vi "Param.vi"() -> ()   [LabVIEW 2015]
uses:
  Variable globale.vi
panel:
  in  "Decel":dbl
  in  "Accel":dbl
  in  "stop":bool
  in  "Ressolution Codeur":dbl
  in  "Diametre Galet Codeur":dbl
  in  "Diametre Plateau":dbl
  in  "Decel Max":dbl
  in  "Accel Max":dbl
  in  "Vitesse Max":dbl
  # "PARAMETRES UTILISATEUR"
  # "mm/s²"
  # "mm/s²"
  # "PARAMETRES SYSTEME"
  # "mm/s"
  # "mm"
  # "mm/s²"
  # "mm"
  # "mm/s²"
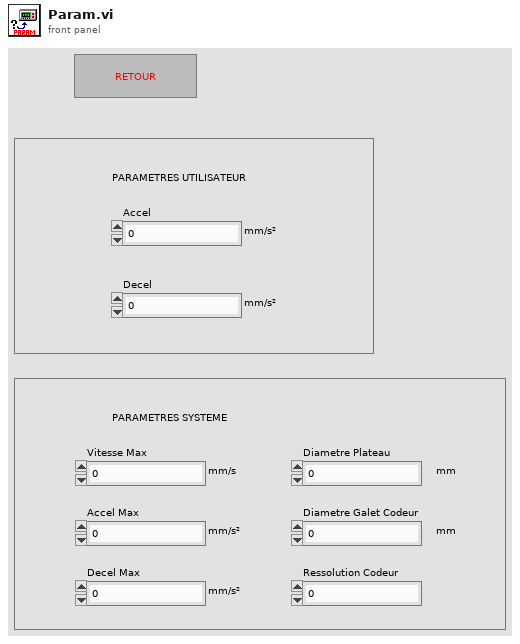
[diagram p1: front panel]
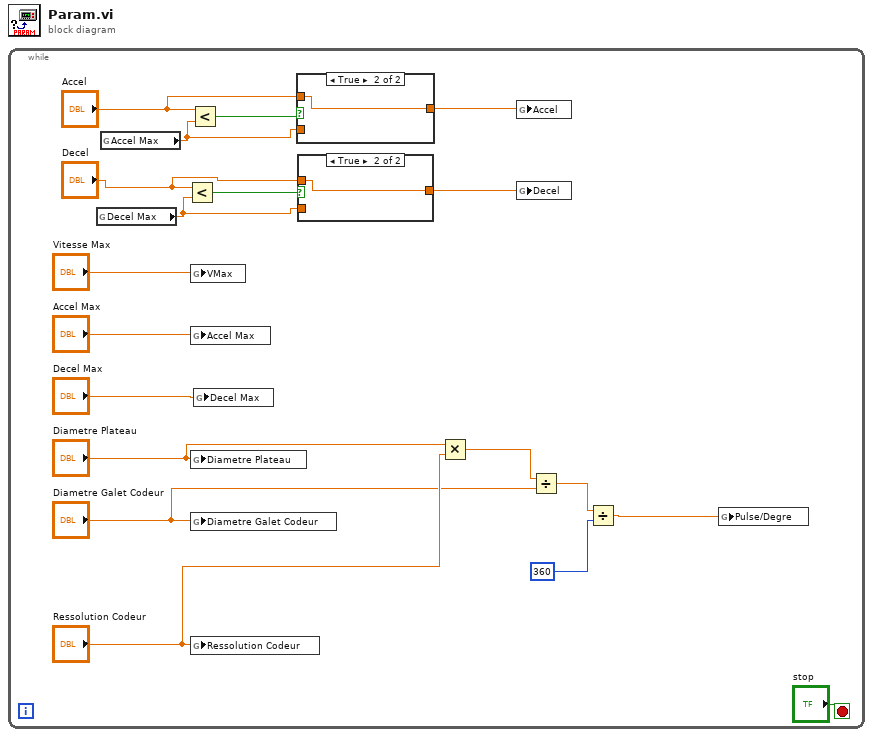
[diagram p0: block diagram]
diagram:
  n1 = while {
    stop <- "stop" stop-if-true
    n2 = global read "Variable globale.vi" "Decel Max"() -> (w2:dbl)
    n3 = global read "Variable globale.vi" "Accel Max"() -> (w6:dbl)
    n4 = Less?(x="Decel", y=w2) -> (x < y?=w4:bool)
    n5 = Less?(x="Accel", y=w6) -> (x < y?=w8:bool)
    n6 = global write "Variable globale.vi" "VMax"("Vitesse Max") -> ()
    n7 = global write "Variable globale.vi" "Accel Max"("Accel Max") -> ()
    n8 = global write "Variable globale.vi" "Diametre Plateau"("Diametre Plateau") -> ()
    n9 = global write "Variable globale.vi" "Diametre Galet Codeur"("Diametre Galet Codeur") -> ()
    n10 = global write "Variable globale.vi" "Ressolution Codeur"("Ressolution Codeur") -> ()
    n11 = global write "Variable globale.vi" "Decel Max"("Decel Max") -> ()
    n12 = case shown="True" w8 {
      tunnel: "Accel" -> [_ w23]
      tunnel: w6 -> [w22 _]
      tunnel: [w22 w23] -> w5
      frame False {
      }
      frame True {
      }
    }
    n13 = case shown="True" w4 {
      tunnel: "Decel" -> [_ w21]
      tunnel: w2 -> [w20 _]
      tunnel: [w20 w21] -> w1
      frame False {
      }
      frame True {
      }
    }
    n14 = Multiply(x="Diametre Plateau", y="Ressolution Codeur") -> (x*y=w14:dbl)
    n15 = global write "Variable globale.vi" "Accel"(w5) -> ()
    n16 = global write "Variable globale.vi" "Decel"(w1) -> ()
    n17 = Divide(x=w14, y="Diametre Galet Codeur") -> (x/y=w12:dbl)
    n18 = Divide(x=w12, y=360) -> (x/y=w10:dbl)
    n19 = global write "Variable globale.vi" "Pulse/Degre"(w10) -> ()
  }
